vi "Discrete CDF.vi"   [LabVIEW 2017, in "NI_Gmath.lvlib"]
doc: "Computes the discrete cumulative distribution function (CDF), or the probability that the random variate X, where X describes the selected distribution type, takes on a value less than or equal to <B>x</B>. You must manually select the polymorphic instance to use."
uses:
  <vilib>/gmath/NI_Gmath.lvlib
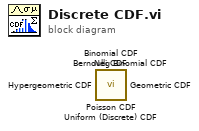
[diagram p0: block diagram]
diagram:
  n1 = call <vilib>:"Poisson CDF.vi"() -> ()  [unwired: 10 in, 2 out]
  n2 = call <vilib>:"Neg Binomial CDF.vi"() -> ()  [unwired: 10 in, 2 out]
  n3 = call <vilib>:"Hypergeometric CDF.vi"() -> ()  [unwired: 10 in, 2 out]
  n4 = call <vilib>:"Geometric CDF.vi"() -> ()  [unwired: 10 in, 2 out]
  n5 = call <vilib>:"Uniform (Discrete) CDF.vi"() -> ()  [unwired: 10 in, 2 out]
  n6 = call <vilib>:"Binomial CDF.vi"() -> ()  [unwired: 10 in, 2 out]
  n7 = call <vilib>:"Bernoulli CDF.vi"() -> ()  [unwired: 10 in, 2 out]
